vi "direct_tcpip.vi"() -> ()   [LabVIEW 2013]
uses:
  libssh2.lvlib
panel:
  in  "stop":bool
  out "error out":errorcluster
  in  "remote_destport":i32=2222
  in  "remote_desthost":string="localhost"
  in  "local_listenport":u16=4444
  in  "local_listenip":string="localhost"
  in  "server_ip":string="127.0.0.1"
  in  "password":string
  in  "username":string
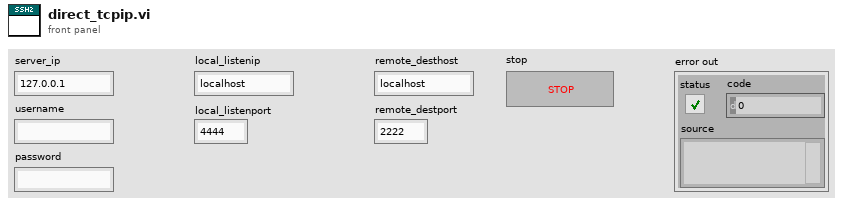
[diagram p1: front panel]
types:
  T1 = enum16{"Standard", "Buffered", "CRLF", "Immediate"}
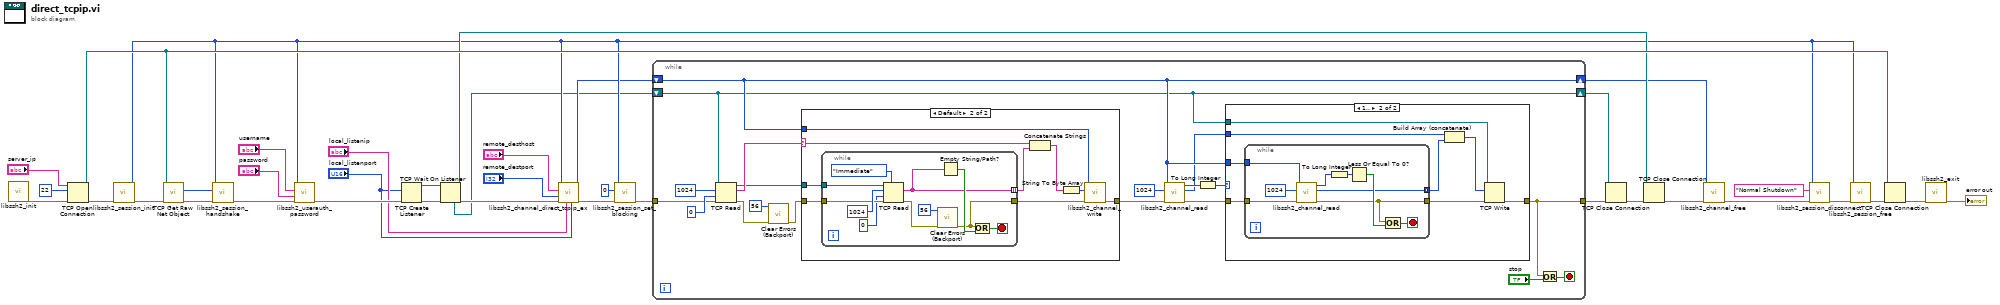
[diagram p0: block diagram]
diagram:
  n1 = call "libssh2_init.vi"() -> ("error out"=w37:errorcluster)  [unwired: 10 in, 1 out]
  n2 = TCP Open Connection(address="server_ip", remote port or service name=u16 22, error in (no error)=w37) -> (connection ID=w18:refnum<k5>, error out=w34:errorcluster)  [unwired: 2 in]
  n3 = call "libssh2_session_init.vi"("error in (no error)"=w34) -> ("error out"=w33:errorcluster, "return value"=w15:u64)  [unwired: 9 in]
  n4 = call <vilib>:"TCP Get Raw Net Object.vi"("error in (no error)"=w33, "connection ID"=w18) -> ("error out"=w31:errorcluster, "raw net object"=w32:u64)  [unwired: 7 in, 1 out]
  n5 = call "libssh2_session_handshake.vi"("error in (no error)"=w31, "socket"=w32, "session"=w15) -> ("error out"=w30:errorcluster)  [unwired: 7 in, 1 out]
  n6 = call "libssh2_userauth_password.vi"("error in (no error)"=w30, "password"="password", "username"="username", "session"=w15) -> ("error out"=w29:errorcluster)  [unwired: 6 in, 1 out]
  n7 = TCP Create Listener(8:w29, 10:"local_listenport") -> (0:w14:errorcluster, 3:w9:refnum<k5>)  [unwired: 3 in, 1 out]
  n8 = TCP Wait On Listener(8:w14, 11:w9) -> (0:w26:errorcluster, 3:w16:refnum<k5>, 4:w2:refnum<k5>)  [unwired: 2 in, 2 out]
  n9 = call "libssh2_channel_direct_tcpip_ex.vi"("sport"="local_listenport", "shost"="local_listenip", "error in (no error)"=w26, "port"="remote_destport", "host"="remote_desthost", "session"=w15) -> ("error out"=w25:errorcluster, "return value"=w5:u64)  [unwired: 4 in]
  n10 = call "libssh2_session_set_blocking.vi"("error in (no error)"=w25, "blocking"=0, "session"=w15) -> ("error out"=w7:errorcluster)  [unwired: 8 in]
  n11 = while {
    tunnel: w7 -> [w45]
    tunnel: [w40] -> w6
    shift-right: [w48] -> w3
    shift-left: w5 -> [w48]
    shift-right: [w42] -> w1
    shift-left: w2 -> [w42]
    stop <- w38 stop-if-true
    n12 = TCP Read(connection ID=w42, bytes to read=1024, error in (no error)=w45, 9:0 ("timeout ms (25000)")) -> (connection ID out=w43:refnum<k5>, data out=w55:string, error out=w47:errorcluster)  [unwired: 1 in]
    n13 = call "Clear Errors (Backport).vi"("error in (no error)"=w47, "specific error code to clear (0: all)"=56) -> ("error out"=w44:errorcluster)  [unwired: 4 in, 1 out]
    n14 = case shown="Default" w55 {
      selector: w55 -> [_ w78]
      tunnel: [w75 w81] -> w51
      tunnel: w43 -> [_ w84]
      tunnel: w44 -> [w75 w83]
      tunnel: w48 -> [_ w80]
      frame "" {
      }
      frame Default {
        n15 = while {
          tunnel: [w86] -> w82
          tunnel: w84 -> [w93]
          tunnel: w83 -> [w90]
          tunnel: [w85] -> w79 mode=indexing
          stop <- w91 stop-if-true
          n16 = TCP Read(connection ID=w93, bytes to read=1024, error in (no error)=w90, 7:T1."Immediate" ("mode (standard)"), 9:0 ("timeout ms (25000)")) -> (data out=w85:string, error out=w87:errorcluster)  [unwired: 1 out]
          n17 = call "Clear Errors (Backport).vi"("error in (no error)"=w87, "specific error code to clear (0: all)"=56) -> ("error out"=w86:errorcluster)  [unwired: 4 in, 1 out]
          n18 = Empty String/Path?(string/path=w85) -> (empty?=w92:bool)
          n19 = Or(x=w86, y=w92) -> (x .or. y?=w91:bool)
        }
        n20 = Concatenate Strings(w78, w79) -> (w77:string)
        n21 = String To Byte Array(string=w77) -> (unsigned byte array=w76:u8[])
        n22 = call "libssh2_channel_write.vi"("error in (no error)"=w82, "buf"=w76, "channel"=w80) -> ("error out"=w81:errorcluster)  [unwired: 7 in, 1 out]
      }
    }
    n23 = call "libssh2_channel_read.vi"("error in (no error)"=w51, "buflen"=u64 1024, "channel"=w48) -> ("error out"=w50:errorcluster, "buf"=w41:u8[], "return value"=w49:u64)  [unwired: 6 in]
    n24 = To Long Integer(number=w49) -> (32bit integer=w53:i32)
    n25 = case shown="1.." w53 {
      tunnel: [w57 w63] -> w40
      tunnel: w48 -> [_ w65]
      tunnel: w42 -> [_ w62]
      tunnel: w50 -> [w57 w64]
      tunnel: w41 -> [_ w61]
      frame Default {
      }
      frame 1.. {
        n26 = while {
          tunnel: w65 -> [w69]
          tunnel: w64 -> [w70]
          tunnel: [w67] -> w60 mode=concatenating
          tunnel: [w66] -> w58
          stop <- w74 stop-if-true
          n27 = call "libssh2_channel_read.vi"("error in (no error)"=w70, "buflen"=u64 1024, "channel"=w69) -> ("error out"=w66:errorcluster, "buf"=w67:u8[], "return value"=w68:u64)  [unwired: 6 in]
          n28 = To Long Integer(number=w68) -> (32bit integer=w72:i32)
          n29 = Less Or Equal To 0?(x=w72) -> (x <= 0?=w73:bool)
          n30 = Compound Arithmetic op=OR(w66, w73) -> (w74:bool)
        }
        n31 = Build Array (concatenate)(w61, w60) -> (w59:u8[])
        n32 = TCP Write(connection ID=w62, data in=w59, error in (no error)=w58) -> (error out=w63:errorcluster)  [unwired: 1 in, 2 out]
      }
    }
    n33 = Or(x=w40, y="stop") -> (x .or. y?=w38:bool)
  }
  n34 = TCP Close Connection(connection ID=w1, error in (no error)=w6) -> (error out=w8:errorcluster)  [unwired: 1 in, 1 out]
  n35 = TCP Close Connection(connection ID=w16, error in (no error)=w8) -> (error out=w20:errorcluster)  [unwired: 1 in, 1 out]
  n36 = call "libssh2_channel_free.vi"("error in (no error)"=w20, "channel"=w3) -> ("error out"=w23:errorcluster)  [unwired: 8 in, 1 out]
  n37 = call "libssh2_session_disconnect.vi"("error in (no error)"=w23, "description"="Normal Shutdown", "session"=w15) -> ("error out"=w21:errorcluster)  [unwired: 7 in, 1 out]
  n38 = call "libssh2_session_free.vi"("error in (no error)"=w21, "session"=w15) -> ("error out"=w19:errorcluster)  [unwired: 8 in, 1 out]
  n39 = TCP Close Connection(connection ID=w18, error in (no error)=w19) -> (error out=w4:errorcluster)  [unwired: 1 in, 1 out]
  n40 = call "libssh2_exit.vi"("error in (no error)"=w4) -> ("error out"=→"error out":errorcluster)  [unwired: 10 in]
